vi "MCSHostTest.vi"() -> ()   [LabVIEW 2014]
uses:
  <vilib>/FPGAPlugInAG/PXI-7852R/niLvFpga_Open_PXI-7852R.vi
  <vilib>/rvi/interface/common/dynamic/niFpgaDynamicAddResources.vi
  <vilib>/rvi/interface/common/niFpgaWaitOnOcc.vi
  <vilib>/Utility/error.llb/Error Cluster From Error Code.vi
  <vilib>/rvi/errors/niLvFpgaAdjustHostInterfaceError.vi
  <vilib>/FPGAPlugInAG/Dynamic/niLvFpga_Close_Dynamic.vi
  <vilib>/rvi/interface/nirviOpenFPGA/nirviOpenFPGA.xnode
  bin/TimeResolvedSequencer/NiFpga_TRS_DAF_104.lvbitx
  <vilib>/rvi/interface/nirviMethod/nirviMethod.xnode
  <vilib>/rvi/interface/nirviReadWriteControl/nirviReadWriteControl.xnode
  <vilib>/rvi/interface/nirviCloseFPGA/nirviCloseFPGA.xnode
  NiFpgaLv.dll
  <vilib>/rvi/interface/Simulation/niFpgaSimulationCallBeginRW.vi
  <vilib>/rvi/errors/niLvFpgaMergeErrorWithErrorCode.vi
  <vilib>/FPGAPlugInAG/Dynamic/niLvFpga_ReadFifo_Dynamic.vi
  <vilib>/FPGAPlugInAG/Dynamic/niLvFpga_ConfigureFifo_Dynamic.vi
panel:
  out "postAccOffsetVoltState":T1(ring)
  in  "postAccOffsetVoltControl":T1(ring)
  in  "triggerTypes":enum16{"noTrigger", "singleHitDelay"}(ring)
  out "TRSArray":u32[][][](array[numeric])
  in  "SendHaltAbort":bool
  out "TRSdataUntouchedOut":u32[](array[numeric]) format="%032b"
  out "VoltArray":u32[](array[numeric]) format="%032b"
  in  "AnalyseData":bool
  out "ReadData":u32[](array[numeric]) format="%032b"
  out "SavedData":u32[](array[numeric]) format="%032b"
  in  "SendCommand":bool
  out "MCSQuWriteTimeout":bool
  out "DACQuWriteTimeout":bool
  out "MCSerrorcount":i8
  in  "cmdByHost":T2(ring)
  out "MCSstate":enum16{"idle", "scanning", "done", "error"}(ring)
  out "seqState":T2(ring)
  in  "nOfBunches":i32
  in  "nOfBins":u32=4000
  in  "delay(ticks)":u32=1000
  in  "MCSSelectTrigger":T3(ring)=enum."Int0"
  in  "hostConfirmsHzOffsetIsSet":bool
  in  "halt":bool
  in  "abort":bool
  in  "measVoltTimeout(10ns)":i32
  in  "measVoltPulseLength(25ns)":i32
  in  "waitAfterReset(25nsTicks)":u16=400
  in  "waitForKepco(25nsTicks)":u16=400
  in  "invertScan":bool
  in  "nOfScans":i32=6
  in  "nOfSteps":i32=6
  in  "start":i32 format="%024b"
  in  "stepSize":i32=2048 format="%024b"
  in  "VoltOrScaler?":bool
  out "measVoltState":T4(ring)
  in  "SetParameters":bool
  in  "stop":bool
  # "cmd is send when control in ui changes"
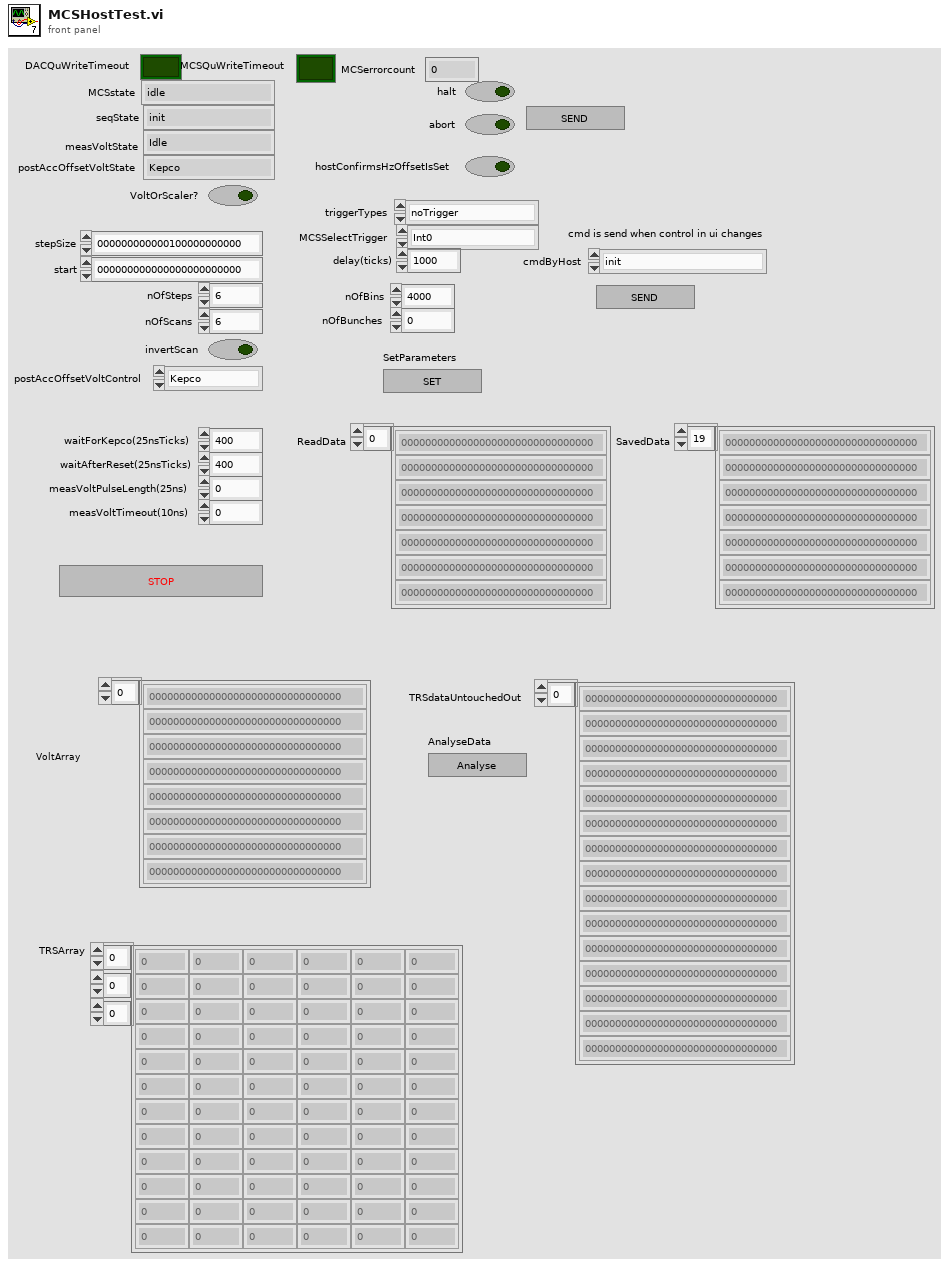
[diagram p1: front panel]
types:
  T1 = enum8{"Kepco", "Heinzinger0", "Heinzinger1", "Heinzinger2", "loading"}
  T2 = enum16{"init", "idle", "measureOffset", "measureTrack", "measComplete", "error"}
  T3 = enum8{"Ext0", "Ext1", "Ext2", "Ext3", "Ext4", "Ext5", "Ext6", "Ext7", "Int0", "Int1", "Int2", "Int3", "Int4", "Int5", "Int6", "Int7"}
  T4 = enum16{"Idle", "sendMeasRequest", "waitUntilDone", "done"}
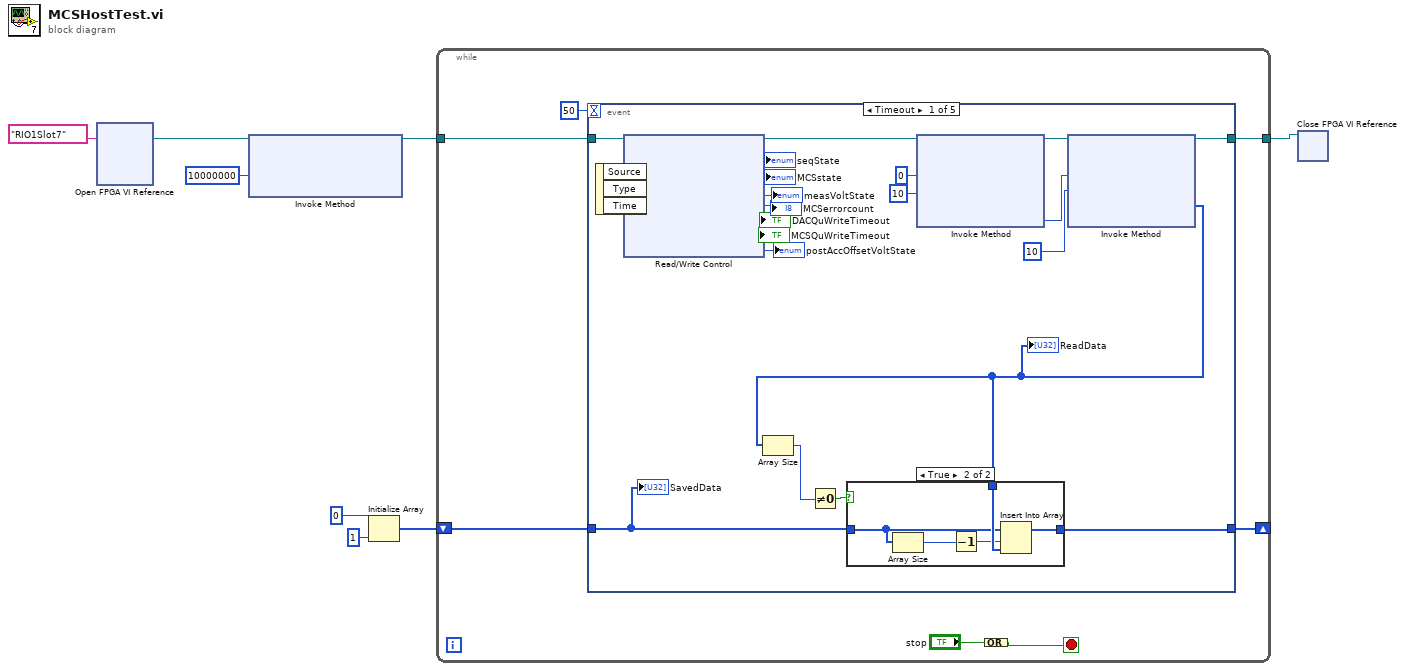
[diagram p0: block diagram]
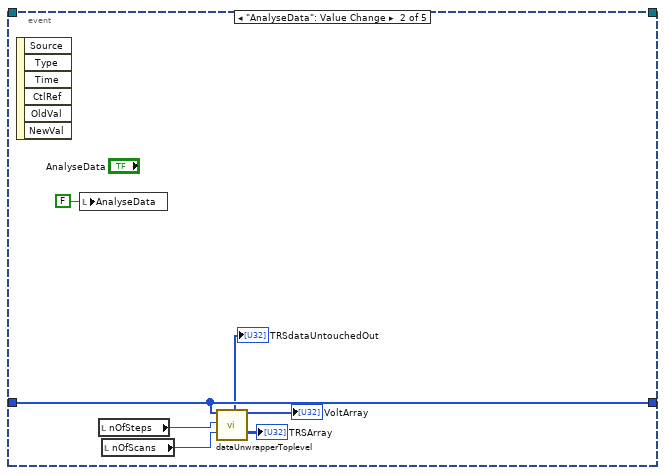
[diagram p3: hidden frame]
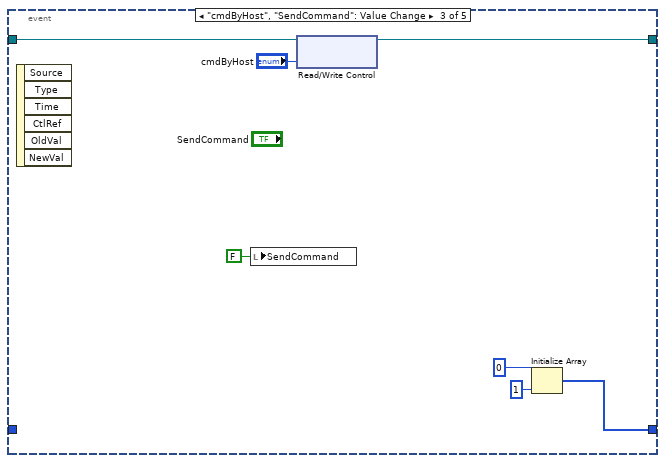
[diagram p4: hidden frame]
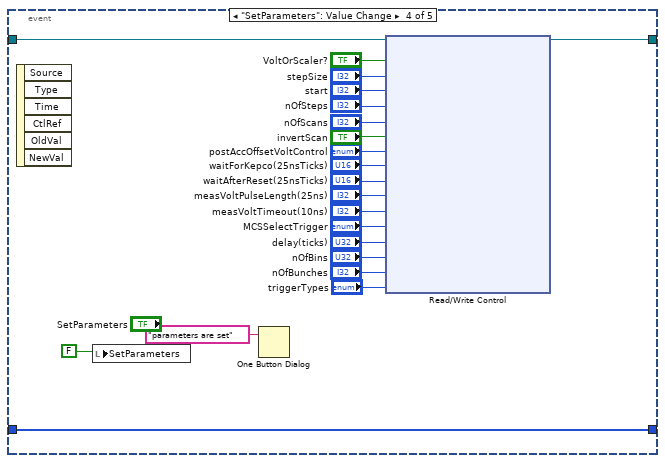
[diagram p5: hidden frame]
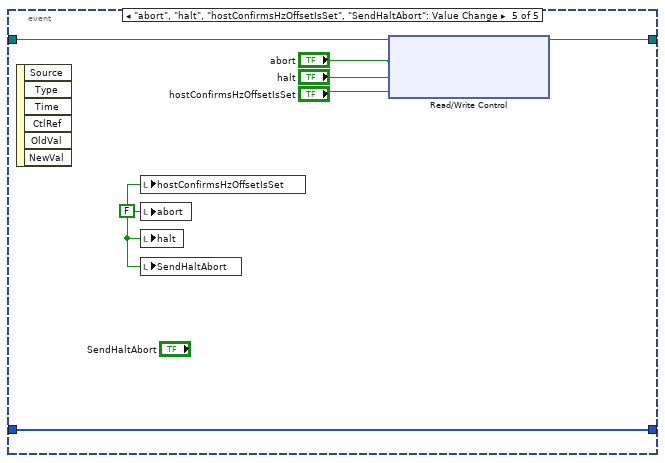
[diagram p6: hidden frame]
diagram:
  n1 = xnode "Open FPGA VI Reference"("resource name"=tag "RIO1Slot7") -> ("FPGA VI Reference Out"=w8:refnum<k20>)  [unwired: 1 in, 1 out]
  n2 = xnode "Invoke Method"("FPGA VI Reference In"=w8, "Requested Depth"=u32 10000000) -> ("FPGA VI Reference Out"=w5:refnum<k20>)  [unwired: 1 in, 2 out]
  n3 = Initialize Array(u32 0 ("element"), 1 ("dimension size")) -> (w1:u32[])
  n4 = while {
    tunnel: w5 -> [w12]
    tunnel: [w11] -> w7
    shift-right: [w10] -> _
    shift-left: w1 -> [w9]
    stop <- w13 stop-if-true
    n5 = event shown="[0] Timeout" {
      selector: _ -> [_ _ _ _ _]
      dyn-events: _ -> [_ _ _ _ _]
      timeout: 50 -> [_ _ _ _ _]
      tunnel: w12 -> [w35 _ w55 w75 w83]
      tunnel: [w29 _ w54 w60 w82] -> w11
      tunnel: [w19 w47 w49 w59 w78] -> w10
      tunnel: w9 -> [w18 w47 _ w59 w78]
      event Timeout {
        n6 = event-data() -> ()  [unwired: 1 in, 3 out]
        n7 = xnode "Read/Write Control"("FPGA VI Reference In"=w35) -> ("FPGA VI Reference Out"=w33:refnum<k20>, "seqState"=→"seqState":T2, "MCSstate"=→"MCSstate":enum16{"idle", "scanning", "done", "error"}, "measVoltState"=→"measVoltState":T4, "MCSerrorcount"=→"MCSerrorcount":i8, "DACQuWriteTimeout"=→"DACQuWriteTimeout":bool, "MCSQuWriteTimeout"=→"MCSQuWriteTimeout":bool, "postAccOffsetVoltState"=→"postAccOffsetVoltState":T1)  [unwired: 1 in, 1 out]
        n8 = xnode "Invoke Method"("FPGA VI Reference In"=w33, "Number of Elements"=u32 0, "Timeout (ms)"=10) -> ("FPGA VI Reference Out"=w32:refnum<k20>, "Elements Remaining"=w28:u32)  [unwired: 1 in, 2 out]
        n9 = xnode "Invoke Method"("FPGA VI Reference In"=w32, "Number of Elements"=w28, "Timeout (ms)"=10) -> ("FPGA VI Reference Out"=w29:refnum<k20>, "Data"=w17:u32[])  [unwired: 1 in, 2 out]
        "ReadData" <- w17
        n10 = Array Size(array=w17) -> (size(s)=w20:i32)
        n11 = Not Equal To 0?(x=w20) -> (x != 0?=w21:bool)
        n12 = case shown="True" w21 {
          tunnel: w17 -> [_ w41]
          tunnel: [w36 w40] -> w19
          tunnel: w18 -> [w36 w39]
          frame False {
          }
          frame True {
            n13 = Array Size(array=w39) -> (size(s)=w38:i32)
            n14 = Decrement(x=w38) -> (x-1=w37:i32)
            n15 = Insert Into Array(array=w39, index=w37, new element=w41) -> (w40:u32[])
          }
        }
        "SavedData" <- w18
      }
      event "AnalyseData": Value Change {
        n16 = event-data() -> ()  [unwired: 1 in, 6 out]
        n17 = local write "AnalyseData"(FALSE ("AnalyseData")) -> ()
        n18 = local read "nOfSteps"() -> (w46:i32)
        n19 = local read "nOfScans"() -> (w45:i32)
        n20 = call "dataUnwrapperToplevel.vi"("dataIn"=w47, "nOfSteps"=w46, "nOfScans"=w45) -> ("DataUntouchedOut"=→"TRSdataUntouchedOut":u32[], "VoltArray"=→"VoltArray":u32[], "TRSArray"=→"TRSArray":u32[][][])  [unwired: 13 in, 1 out]
      }
      event "cmdByHost", "SendCommand": Value Change {
        n21 = event-data() -> ()  [unwired: 1 in, 6 out]
        n22 = local write "SendCommand"(FALSE ("SendCommand")) -> ()
        n23 = xnode "Read/Write Control"("FPGA VI Reference In"=w55, "cmdByHost"="cmdByHost") -> ("FPGA VI Reference Out"=w54:refnum<k20>)  [unwired: 1 in, 1 out]
        n24 = Initialize Array(u32 0 ("element"), 1 ("dimension size")) -> (w49:u32[])
      }
      event "SetParameters": Value Change {
        n25 = event-data() -> ()  [unwired: 1 in, 6 out]
        n26 = local write "SetParameters"(FALSE ("SetParameters")) -> ()
        n27 = One Button Dialog(message="parameters are set") -> ()  [unwired: 1 in, 1 out]
        n28 = xnode "Read/Write Control"("FPGA VI Reference In"=w75, "VoltOrScaler?"="VoltOrScaler?", "dacStepSize18Bit"="stepSize", "dacStartRegister18Bit"="start", "nOfSteps"="nOfSteps", "nOfScans"="nOfScans", "invertScan"="invertScan", "postAccOffsetVoltControl"="postAccOffsetVoltControl", "waitForKepco(25nsTicks)"="waitForKepco(25nsTicks)", "waitAfterReset(25nsTicks)"="waitAfterReset(25nsTicks)", "measVoltPulseLength(25ns)"="measVoltPulseLength(25ns)", "measVoltTimeout(10ns)"="measVoltTimeout(10ns)", "selectTrigger"="MCSSelectTrigger", "delay_10ns_ticks"="delay(ticks)", "nOfBins"="nOfBins", "nOfBunches"="nOfBunches", "triggerTypes"="triggerTypes") -> ("FPGA VI Reference Out"=w60:refnum<k20>)  [unwired: 1 in, 1 out]
      }
      event "abort", "halt", "hostConfirmsHzOffsetIsSet", "SendHaltAbort": Value Change {
        w77 = FALSE ("abort")
        n29 = event-data() -> ()  [unwired: 1 in, 6 out]
        n30 = local write "hostConfirmsHzOffsetIsSet"(w77) -> ()
        n31 = local write "abort"(w77) -> ()
        n32 = local write "halt"(w77) -> ()
        n33 = local write "SendHaltAbort"(w77) -> ()
        n34 = xnode "Read/Write Control"("FPGA VI Reference In"=w83, "abort"="abort", "halt"="halt", "hostConfirmsHzOffsetIsSet"="hostConfirmsHzOffsetIsSet") -> ("FPGA VI Reference Out"=w82:refnum<k20>)  [unwired: 1 in, 1 out]
      }
    }
    n35 = Compound Arithmetic op=OR("stop") -> (w13:bool)
  }
  n36 = xnode "Close FPGA VI Reference"("FPGA VI Reference In"=w7) -> ()  [unwired: 1 in, 1 out]
